vi "SEK2020v1VI8EncontrarTubo.vi"(0 "Parâmetros 2":T1={"Azul Max EV3 Cor"=17, "Azul Min EV3 Cor"=0, "Verde Max EV3 Cor"=6, "Verde Min EV3 Cor"=0, "Vermelho Max Ev3 Cor"=0, "Vermelho Min EV3 Cor"=0, "Chão EV3 Cor"=0.0, "Branco Max EV3 Cor"=0.0, "Branco Min EV3 Cor"=0.0, "Preto Max EV3 Cor"=0.0, "Preto Min EV3 Cor"=0.0, "Distância Tubulação"=0.0, "Distância Frontal"=0.0, "Amarelo Max EV3 Cor"=0.0, "Amarelo Min EV3 Cor"=0.0, "Distância Lateral"=0.0, "90°"=0.0, "180°"=0.0, "Seguidor de Linha"=0.0}, 1 "NXT/EV3":T2, 2 "cor":i32) -> (8 "NXT/EV3 2":T2, 9 "CASE":i32)   [LabVIEW 2016]
uses:
  <vilib>/NXT/Subs/LVHSConnector.ctl
  <vilib>/NXT/LegoClasses/BrickReference/BrickReference.lvclass
  <vilib>/NXT/Block Support/NXT_InputPort.ctl
  <vilib>/NXT/Block Support/NXT_OutputPort.ctl
  <vilib>/NXT/Dual Mode Library/Sensors/EV3_Ultrasonic_CM.vi
  <vilib>/NXT/Dual Mode Library/Sensors/EV3_Color_Reflect.vi
  <vilib>/NXT/NXTIO Xnodes/NXTIONodeSubVIs/NXTStopMotors.vi
  <vilib>/NXT/NXTIO Xnodes/NXTIONodeSubVIs/NXTMoveMotors.vi
  <vilib>/NXT/NXTIO Xnodes/AddressXNode/NXTIOAddress.xnode
  <vilib>/NXT/NXTIO Xnodes/NXTIOXNode/NXTIO.xnode
panel:
  # "Sensor EV3 Cor"
  # "Sensor Ultrassônico"
  # "Sensor Giroscópio"
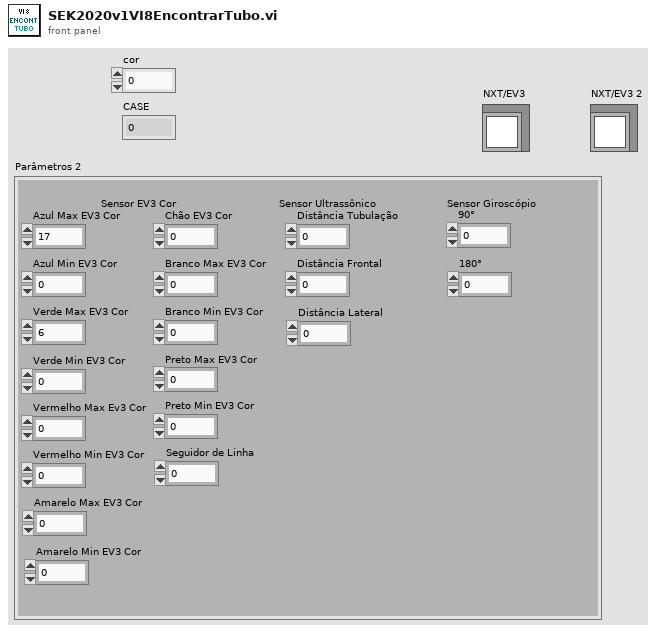
[diagram p1: front panel]
types:
  T1 = cluster{"Azul Max EV3 Cor":i32, "Azul Min EV3 Cor":i32, "Verde Max EV3 Cor":i32, "Verde Min EV3 Cor":i32, "Vermelho Max Ev3 Cor":i32, "Vermelho Min EV3 Cor":i32, "Chão EV3 Cor":sgl, "Branco Max EV3 Cor":sgl, "Branco Min EV3 Cor":sgl, "Preto Max EV3 Cor":sgl, "Preto Min EV3 Cor":sgl, "Distância Tubulação":sgl, "Distância Frontal":sgl, "Amarelo Max EV3 Cor":dbl, "Amarelo Min EV3 Cor":dbl, "Distância Lateral":sgl, "90°":sgl, "180°":sgl, "Seguidor de Linha":dbl}
  T2 = typedef "LVHSConnector.ctl" = refnum<class "BrickReference.lvclass">
  T3 = typedef "NXT_OutputPort.ctl" = u8
  T4 = typedef "NXT_InputPort.ctl" = u32
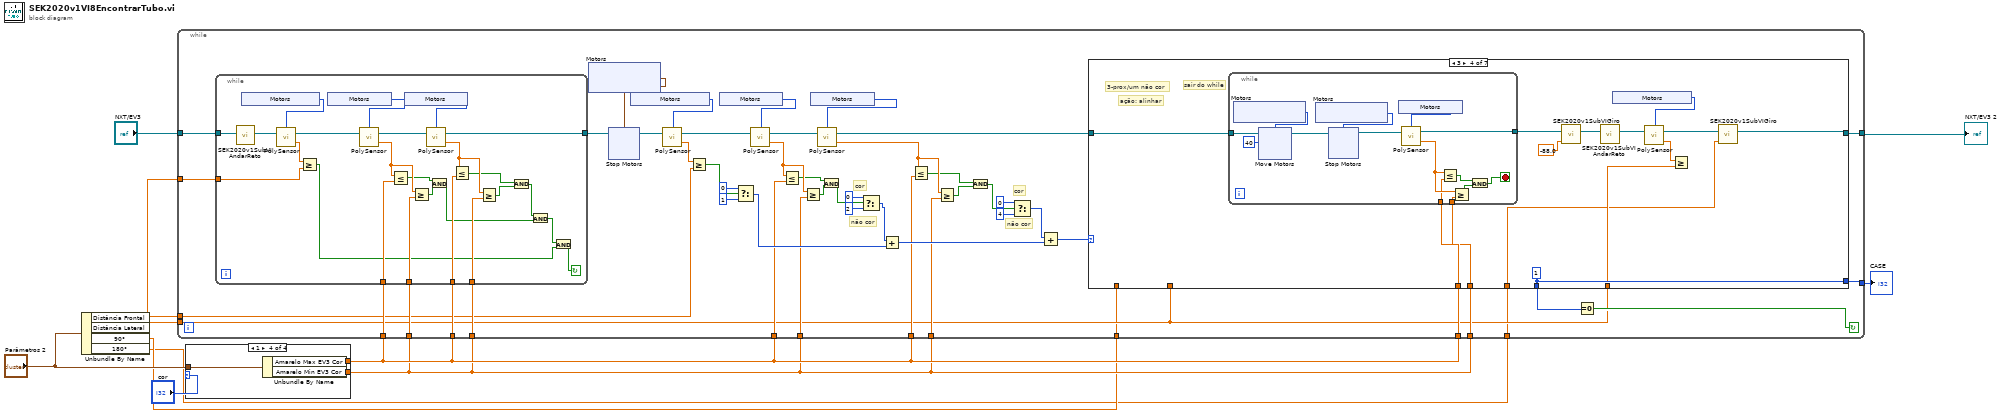
[diagram p0: block diagram]
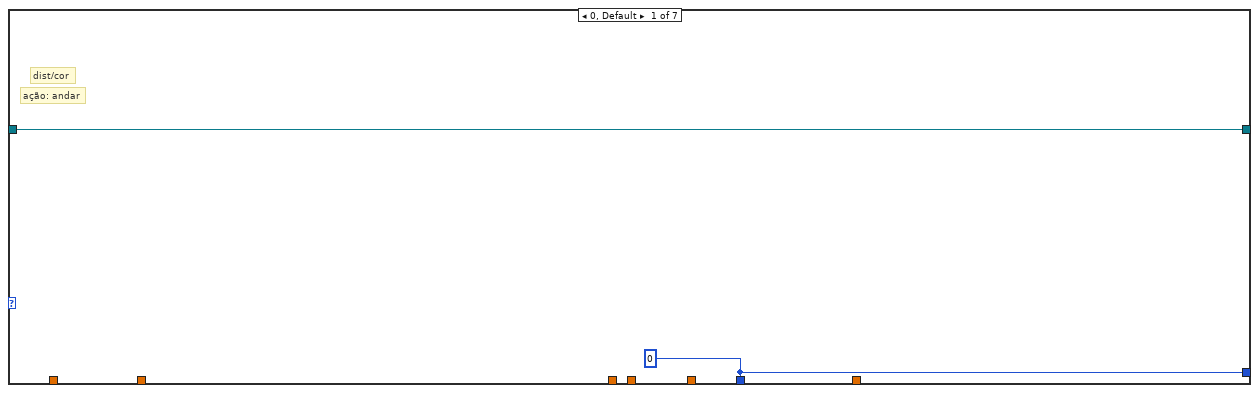
[diagram p2: hidden frame]
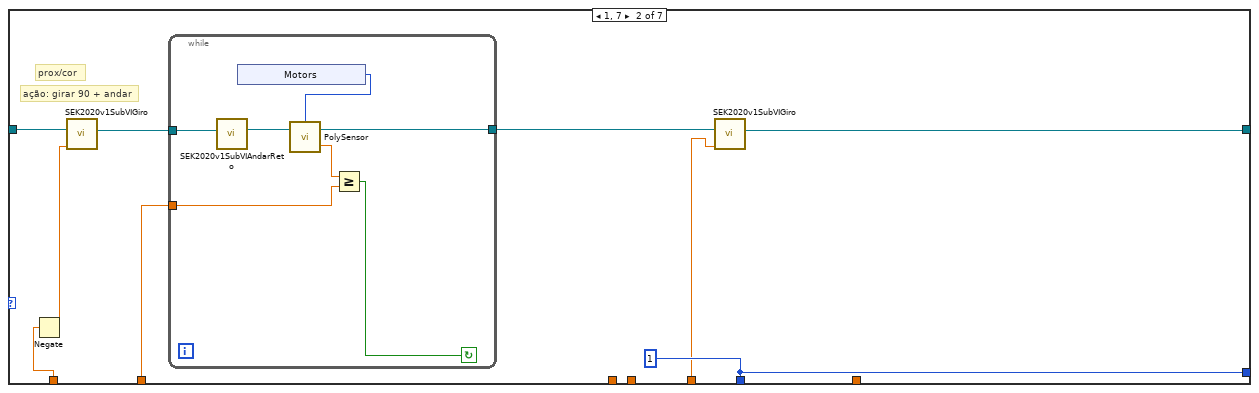
[diagram p3: hidden frame]
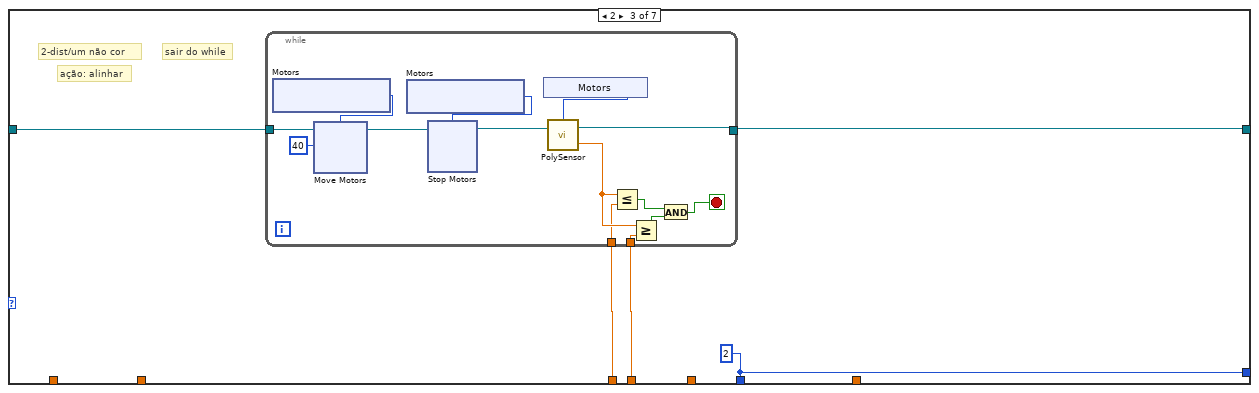
[diagram p4: hidden frame]
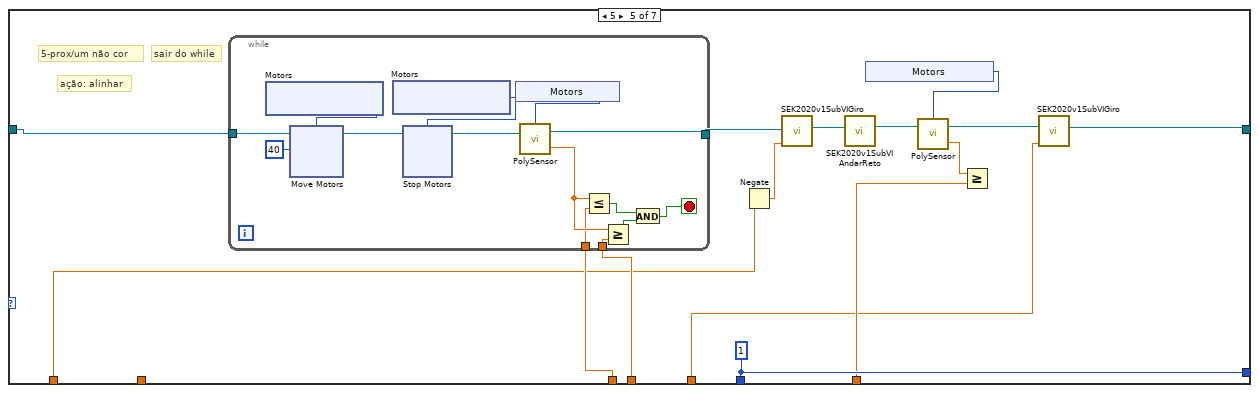
[diagram p5: hidden frame]
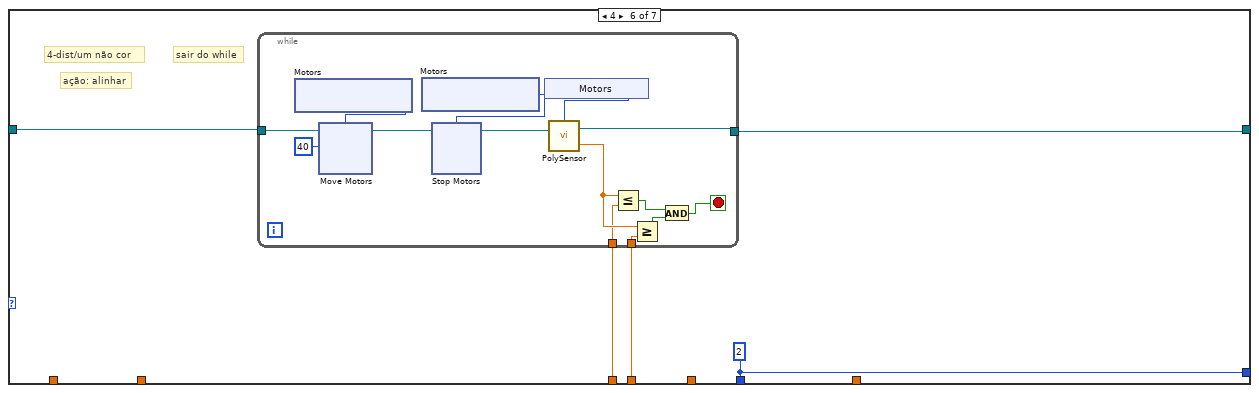
[diagram p6: hidden frame]
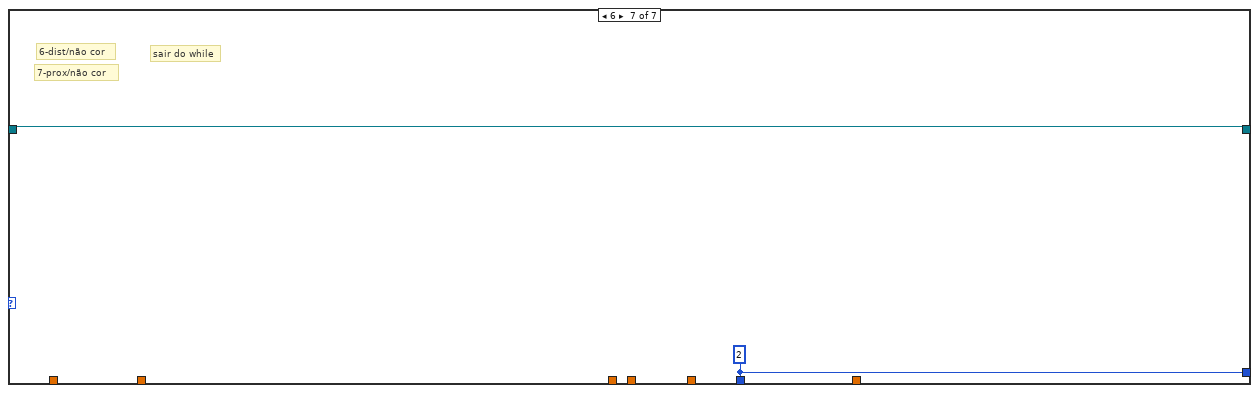
[diagram p7: hidden frame]
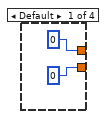
[diagram p8: hidden frame]
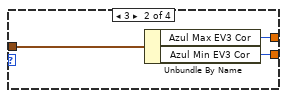
[diagram p9: hidden frame]
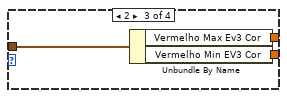
[diagram p10: hidden frame]
diagram:
  n1 = Unbundle By Name("Parâmetros 2") -> ("Distância Frontal"=w6:sgl, "Distância Lateral"=w5:sgl, "90°"=w2:sgl, "180°"=w1:sgl)
  n2 = case shown="1" "cor" {
    tunnel: "Parâmetros 2" -> [_ w16 w19 w22]
    tunnel: [0 w15 w18 w21] -> w8
    tunnel: [0 w14 w17 w20] -> w7
    frame Default {
    }
    frame 3 {
      n3 = Unbundle By Name(w16) -> ("Azul Max EV3 Cor"=w15:i32, "Azul Min EV3 Cor"=w14:i32)
    }
    frame 2 {
      n4 = Unbundle By Name(w19) -> ("Vermelho Max Ev3 Cor"=w18:i32, "Vermelho Min EV3 Cor"=w17:i32)
    }
    frame 1 {
      n5 = Unbundle By Name(w22) -> ("Amarelo Max EV3 Cor"=w21:dbl, "Amarelo Min EV3 Cor"=w20:dbl)
    }
  }
  n6 = while {
    tunnel: [w48] -> w4
    tunnel: [w46] -> w10
    tunnel: "NXT/EV3" -> [w45]
    tunnel: w8 -> [w44]
    tunnel: w7 -> [w43]
    tunnel: w8 -> [w42]
    tunnel: w7 -> [w41]
    tunnel: w8 -> [w40]
    tunnel: w8 -> [w39]
    tunnel: w7 -> [w38]
    tunnel: w7 -> [w37]
    tunnel: w8 -> [w36]
    tunnel: w7 -> [w35]
    tunnel: w6 -> [w34]
    tunnel: w6 -> [w33]
    tunnel: w5 -> [w27]
    tunnel: w2 -> [w24]
    tunnel: w1 -> [w23]
    stop <- w49 continue-if-true
    # "não cor"
    # "cor"
    # "não cor"
    # "cor"
    n7 = while {
      tunnel: w34 -> [w97]
      tunnel: w44 -> [w93]
      tunnel: w43 -> [w91]
      tunnel: w42 -> [w90]
      tunnel: w41 -> [w88]
      tunnel: [w79] -> w26
      tunnel: w45 -> [w78]
      stop <- w80 continue-if-true
      n8 = call "SEK2020v1SubVIAndarReto.vi"("NXT/EV3"=w78) -> ("NXT/EV3 2"=w77:T2)  [unwired: 9 in]
      n9 = xnode "Motors"() -> ("Sensor"=w76:T4)
      n10 = call-poly <vilib>:"PolySensor.vi"("NXT/EV3"=w77, "Port (Port 1)"=w76) -> ("Centimeters"=w75:sgl, "NXT/EV3"=w73:T2)  [unwired: 1 in]
      n11 = Greater Or Equal?(x=w75, y=w97) -> (x >= y?=w74:bool)
      n12 = xnode "Motors"() -> ("Sensor"=w96:T4)
      n13 = call-poly <vilib>:"PolySensor.vi"("NXT/EV3"=w73, "Port (Port 1)"=w96) -> ("Scaled Value"=w92:sgl, "NXT/EV3"=w94:T2)  [unwired: 1 in]
      n14 = Less Or Equal?(x=w92, y=w93) -> (x <= y?=w86:bool)
      n15 = xnode "Motors"() -> ("Sensor"=w95:T4)
      n16 = Greater Or Equal?(x=w92, y=w91) -> (x >= y?=w87:bool)
      n17 = call-poly <vilib>:"PolySensor.vi"("NXT/EV3"=w94, "Port (Port 1)"=w95) -> ("Scaled Value"=w89:sgl, "NXT/EV3"=w79:T2)  [unwired: 1 in]
      n18 = And(x=w86, y=w87) -> (x .and. y?=w83:bool)
      n19 = Less Or Equal?(x=w89, y=w90) -> (x <= y?=w84:bool)
      n20 = Greater Or Equal?(x=w89, y=w88) -> (x >= y?=w85:bool)
      n21 = And(x=w84, y=w85) -> (x .and. y?=w82:bool)
      n22 = And(x=w82, y=w83) -> (x .and. y?=w81:bool)
      n23 = And(x=w81, y=w74) -> (x .and. y?=w80:bool)
    }
    n24 = xnode "Motors"() -> ("Motor"=w32:cluster{"Port":T3, "Port":T3})
    n25 = xnode "Stop Motors"("Motors"=w32, "NXT/EV3"=w26) -> ("NXT/EV3"=w31:T2)
    n26 = xnode "Motors"() -> ("Sensor"=w72:T4)
    n27 = call-poly <vilib>:"PolySensor.vi"("NXT/EV3"=w31, "Port (Port 1)"=w72) -> ("Centimeters"=w71:sgl, "NXT/EV3"=w70:T2)  [unwired: 1 in]
    n28 = Greater Or Equal?(x=w71, y=w33) -> (x >= y?=w59:bool)
    n29 = xnode "Motors"() -> ("Sensor"=w69:T4)
    n30 = Select(t=0, s=w59, f=1) -> (s? t:f=w51:i32)
    n31 = call-poly <vilib>:"PolySensor.vi"("NXT/EV3"=w70, "Port (Port 1)"=w69) -> ("Scaled Value"=w66:sgl, "NXT/EV3"=w67:T2)  [unwired: 1 in]
    n32 = Less Or Equal?(x=w66, y=w40) -> (x <= y?=w63:bool)
    n33 = Greater Or Equal?(x=w66, y=w38) -> (x >= y?=w64:bool)
    n34 = xnode "Motors"() -> ("Sensor"=w68:T4)
    n35 = call-poly <vilib>:"PolySensor.vi"("NXT/EV3"=w67, "Port (Port 1)"=w68) -> ("Scaled Value"=w65:sgl, "NXT/EV3"=w25:T2)  [unwired: 1 in]
    n36 = And(x=w63, y=w64) -> (x .and. y?=w60:bool)
    n37 = Select(t=0, s=w60, f=2) -> (s? t:f=w29:i32)
    n38 = Add(x=w29, y=w51) -> (x+y=w50:i32)
    n39 = Less Or Equal?(x=w65, y=w39) -> (x <= y?=w61:bool)
    n40 = Greater Or Equal?(x=w65, y=w37) -> (x >= y?=w62:bool)
    n41 = And(x=w61, y=w62) -> (x .and. y?=w52:bool)
    n42 = Select(t=0, s=w52, f=4) -> (s? t:f=w28:i32)
    n43 = Add(x=w28, y=w50) -> (x+y=w30:i32)
    n44 = case shown="3" w30 {
      tunnel: w25 -> [w108 w117 w128 w172 w207 w251 w283]
      tunnel: [w108 w114 w129 w162 w212 w252 w283] -> w48
      tunnel: [w107 w113 w130 w173 w218 w253 w284] -> w47
      tunnel: [w107 w113 w130 w173 w218 w253 w284] -> w46
      tunnel: w36 -> [_ _ w127 w171 w209 w250 _]
      tunnel: w35 -> [_ _ w126 w170 w208 w249 _]
      tunnel: w27 -> [_ w112 _ _ _ _ _]
      tunnel: w27 -> [_ _ _ w161 w211 _ _]
      tunnel: w24 -> [_ w111 _ _ w206 _ _]
      tunnel: w23 -> [_ w109 _ w160 w204 _ _]
      frame 0, Default {
        w107 = 0
        # "ação: andar"
        # "dist/cor"
      }
      frame 1, 7 {
        w113 = 1
        # "ação: girar 90 + andar"
        # "prox/cor"
        n45 = Negate(x=w111) -> (-x=w110:sgl)
        n46 = call "SEK2020v1SubVIGiro.vi"("ANGULO"=w110, "NXT/EV3"=w117) -> ("NXT/EV3 2"=w116:T2)  [unwired: 7 in]
        n47 = while {
          tunnel: w112 -> [w122]
          tunnel: w116 -> [w121]
          tunnel: [w118] -> w115
          stop <- w120 continue-if-true
          n48 = call "SEK2020v1SubVIAndarReto.vi"("NXT/EV3"=w121) -> ("NXT/EV3 2"=w124:T2)  [unwired: 9 in]
          n49 = xnode "Motors"() -> ("Sensor"=w123:T4)
          n50 = call-poly <vilib>:"PolySensor.vi"("NXT/EV3"=w124, "Port (Port 1)"=w123) -> ("Centimeters"=w119:sgl, "NXT/EV3"=w118:T2)  [unwired: 1 in]
          n51 = Greater Or Equal?(x=w119, y=w122) -> (x >= y?=w120:bool)
        }
        n52 = call "SEK2020v1SubVIGiro.vi"("ANGULO"=w109, "NXT/EV3"=w115) -> ("NXT/EV3 2"=w114:T2)  [unwired: 7 in]
      }
      frame 2 {
        w130 = 2
        # "sair do while"
        # "ação: alinhar"
        # "2-dist/um não cor"
        n53 = while {
          tunnel: w128 -> [w143]
          tunnel: [w137] -> w129
          tunnel: w127 -> [w135]
          tunnel: w126 -> [w134]
          stop <- w136 stop-if-true
          n54 = xnode "Motors"() -> ("Motor"=w144:T3)
          n55 = xnode "Move Motors"("Power/Speed 1"=i8 40, "Motors"=w144, "NXT/EV3"=w143) -> ("NXT/EV3"=w133:T2)
          n56 = xnode "Motors"() -> ("Motor"=w131:T3)
          n57 = xnode "Stop Motors"("Motors"=w131, "NXT/EV3"=w133) -> ("NXT/EV3"=w132:T2)
          n58 = xnode "Motors"() -> ("Sensor"=w141:T4)
          n59 = call-poly <vilib>:"PolySensor.vi"("NXT/EV3"=w132, "Port (Port 1)"=w141) -> ("Scaled Value"=w140:sgl, "NXT/EV3"=w137:T2)  [unwired: 1 in]
          n60 = Less Or Equal?(x=w140, y=w135) -> (x <= y?=w138:bool)
          n61 = Greater Or Equal?(x=w140, y=w134) -> (x >= y?=w139:bool)
          n62 = And(x=w138, y=w139) -> (x .and. y?=w136:bool)
        }
      }
      frame 3 {
        w173 = 1
        # "3-prox/um não cor"
        # "sair do while"
        # "ação: alinhar"
        n63 = while {
          tunnel: w172 -> [w186]
          tunnel: [w180] -> w165
          tunnel: w171 -> [w178]
          tunnel: w170 -> [w177]
          stop <- w179 stop-if-true
          n64 = xnode "Motors"() -> ("Motor"=w187:T3)
          n65 = xnode "Move Motors"("Power/Speed 1"=i8 40, "Motors"=w187, "NXT/EV3"=w186) -> ("NXT/EV3"=w176:T2)
          n66 = xnode "Motors"() -> ("Motor"=w174:T3)
          n67 = xnode "Stop Motors"("Motors"=w174, "NXT/EV3"=w176) -> ("NXT/EV3"=w175:T2)
          n68 = xnode "Motors"() -> ("Sensor"=w184:T4)
          n69 = call-poly <vilib>:"PolySensor.vi"("NXT/EV3"=w175, "Port (Port 1)"=w184) -> ("Scaled Value"=w183:sgl, "NXT/EV3"=w180:T2)  [unwired: 1 in]
          n70 = Less Or Equal?(x=w183, y=w178) -> (x <= y?=w181:bool)
          n71 = Greater Or Equal?(x=w183, y=w177) -> (x >= y?=w182:bool)
          n72 = And(x=w181, y=w182) -> (x .and. y?=w179:bool)
        }
        n73 = call "SEK2020v1SubVIGiro.vi"("ANGULO"=sgl -88.0 ("angle"), "NXT/EV3"=w165) -> ("NXT/EV3 2"=w164:T2)  [unwired: 7 in]
        n74 = call "SEK2020v1SubVIAndarReto.vi"("NXT/EV3"=w164) -> ("NXT/EV3 2"=w168:T2)  [unwired: 9 in]
        n75 = xnode "Motors"() -> ("Sensor"=w167:T4)
        n76 = call-poly <vilib>:"PolySensor.vi"("NXT/EV3"=w168, "Port (Port 1)"=w167) -> ("Centimeters"=w166:sgl, "NXT/EV3"=w163:T2)  [unwired: 1 in]
        n77 = Greater Or Equal?(x=w166, y=w161) -> ()  [unwired: 1 out]
        n78 = call "SEK2020v1SubVIGiro.vi"("ANGULO"=w160, "NXT/EV3"=w163) -> ("NXT/EV3 2"=w162:T2)  [unwired: 7 in]
      }
      frame 5 {
        w218 = 1
        # "5-prox/um não cor"
        # "sair do while"
        # "ação: alinhar"
        n79 = while {
          tunnel: [w226] -> w210
          tunnel: w209 -> [w221]
          tunnel: w208 -> [w220]
          tunnel: w207 -> [w219]
          stop <- w225 stop-if-true
          n80 = xnode "Motors"() -> ("Motor"=w232:T3)
          n81 = xnode "Move Motors"("Power/Speed 1"=i8 40, "Motors"=w232, "NXT/EV3"=w219) -> ("NXT/EV3"=w224:T2)
          n82 = xnode "Motors"() -> ("Motor"=w223:T3)
          n83 = xnode "Stop Motors"("Motors"=w223, "NXT/EV3"=w224) -> ("NXT/EV3"=w222:T2)
          n84 = xnode "Motors"() -> ("Sensor"=w230:T4)
          n85 = call-poly <vilib>:"PolySensor.vi"("NXT/EV3"=w222, "Port (Port 1)"=w230) -> ("Scaled Value"=w229:sgl, "NXT/EV3"=w226:T2)  [unwired: 1 in]
          n86 = Less Or Equal?(x=w229, y=w221) -> (x <= y?=w227:bool)
          n87 = Greater Or Equal?(x=w229, y=w220) -> (x >= y?=w228:bool)
          n88 = And(x=w227, y=w228) -> (x .and. y?=w225:bool)
        }
        n89 = Negate(x=w206) -> (-x=w205:sgl)
        n90 = call "SEK2020v1SubVIGiro.vi"("ANGULO"=w205, "NXT/EV3"=w210) -> ("NXT/EV3 2"=w214:T2)  [unwired: 7 in]
        n91 = call "SEK2020v1SubVIAndarReto.vi"("NXT/EV3"=w214) -> ("NXT/EV3 2"=w217:T2)  [unwired: 9 in]
        n92 = xnode "Motors"() -> ("Sensor"=w216:T4)
        n93 = call-poly <vilib>:"PolySensor.vi"("NXT/EV3"=w217, "Port (Port 1)"=w216) -> ("Centimeters"=w215:sgl, "NXT/EV3"=w213:T2)  [unwired: 1 in]
        n94 = Greater Or Equal?(x=w215, y=w211) -> ()  [unwired: 1 out]
        n95 = call "SEK2020v1SubVIGiro.vi"("ANGULO"=w204, "NXT/EV3"=w213) -> ("NXT/EV3 2"=w212:T2)  [unwired: 7 in]
      }
      frame 4 {
        w253 = 2
        # "sair do while"
        # "ação: alinhar"
        # "4-dist/um não cor"
        n96 = while {
          tunnel: w251 -> [w266]
          tunnel: [w260] -> w252
          tunnel: w250 -> [w258]
          tunnel: w249 -> [w257]
          stop <- w259 stop-if-true
          n97 = xnode "Motors"() -> ("Motor"=w267:T3)
          n98 = xnode "Move Motors"("Power/Speed 1"=i8 40, "Motors"=w267, "NXT/EV3"=w266) -> ("NXT/EV3"=w256:T2)
          n99 = xnode "Motors"() -> ("Motor"=w255:T3)
          n100 = xnode "Stop Motors"("Motors"=w255, "NXT/EV3"=w256) -> ("NXT/EV3"=w254:T2)
          n101 = xnode "Motors"() -> ("Sensor"=w264:T4)
          n102 = call-poly <vilib>:"PolySensor.vi"("NXT/EV3"=w254, "Port (Port 1)"=w264) -> ("Scaled Value"=w263:sgl, "NXT/EV3"=w260:T2)  [unwired: 1 in]
          n103 = Less Or Equal?(x=w263, y=w258) -> (x <= y?=w261:bool)
          n104 = Greater Or Equal?(x=w263, y=w257) -> (x >= y?=w262:bool)
          n105 = And(x=w261, y=w262) -> (x .and. y?=w259:bool)
        }
      }
      frame 6 {
        w284 = 2
        # "7-prox/não cor"
        # "sair do while"
        # "6-dist/não cor"
      }
    }
    n106 = Equal To 0?(x=w47) -> (x = 0?=w49:bool)
  }
  "NXT/EV3 2" <- w4
  "CASE" <- w10
